vi "RegisterTimerEvent.vi"(4 "timer task name":string, 5 "interval (sec)":dbl, 6 "type":T1, 7 "process name":string, 8 "error in (no error)":errorcluster, 9 "callback value":variant, 10 "callback action":string, 11 "qbus in":refnum<class "Qbus.lvclass">) -> (0 "error out":errorcluster, 3 "qbus out":refnum<class "Qbus.lvclass">)   [LabVIEW 2017, in "TimerProcess.lvlib"]
doc: "Registers an event with the Timer process. When the event timer expires, the timer sends the callback action and value to the specified process."
uses:
  <vilib>/addons/TimerProcess/TimerProcess.lvlib
  <vilib>/addons/Qbus/Qbus.lvclass
  <vilib>/addons/TimerProcess/controls/taskType.ctl
  <vilib>/addons/TimerProcess/controls/internalTask.ctl
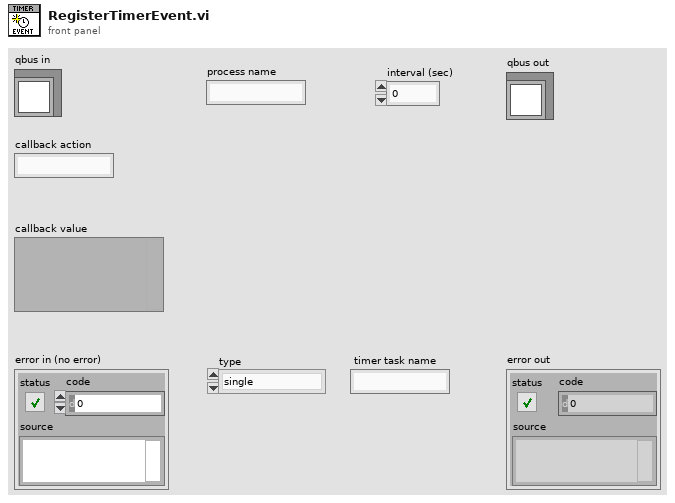
[diagram p1: front panel]
types:
  T1 = typedef "TimerProcess.lvlib/taskType.ctl" = enum16{"single", "repeat"}
  T2 = typedef "TimerProcess.lvlib/internalTask.ctl" = cluster{"Name":string, "Qbus":refnum<class "Qbus.lvclass">, "ProcessName":string, "CallBackAction":string, "CallBackValue":variant, "interval (ms)":i32, "type":T1, "state":cluster{"tickCount":u32}}
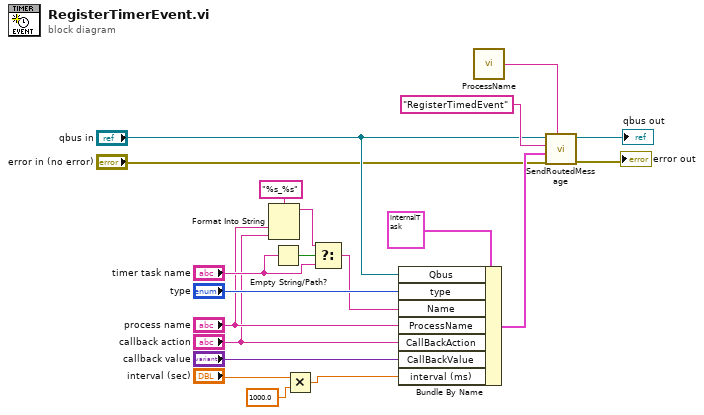
[diagram p0: block diagram]
diagram:
  n1 = Format Into String(format string="%s_%s", "process name", "callback action") -> (resulting string=w1:string)  [unwired: 2 in, 1 out]
  n2 = Empty String/Path?(string/path="timer task name") -> (empty?=w7:bool)
  n3 = Multiply(x="interval (sec)", y=1000.0) -> (x*y=w8:dbl)
  n4 = Select(t=w1, s=w7, f="timer task name") -> (s? t:f=w5:string)
  n5 = Bundle By Name(cluster=T2 {"Name"="", "Qbus"=refnum, "ProcessName"="", "CallBackAction"="", "CallBackValue"=variant, "interval (ms)"=0, "type"=enum."single", "state"={"tickCount"=0}} ("state"), "Qbus"="qbus in", "type"="type", "Name"=w5, "ProcessName"="process name", "CallBackAction"="callback action", "CallBackValue"="callback value", "interval (ms)"=w8) -> (w14:T2)
  n6 = call <vilib>:"ProcessName.vi"() -> ("process name"=w18:string)  [unwired: 5 in]
  n7 = call <vilib>:"SendRoutedMessage.vi"("listener process"=w18, "error in (no error)"="error in (no error)", "message value"=w14, "message name"="RegisterTimedEvent" ("MsgName"), "Qbus in"="qbus in") -> ("error in (no error)"=→"error out":errorcluster, "Qbus out"=→"qbus out":refnum<class "Qbus.lvclass">)  [unwired: 5 in]
